vi "AlmostEqual.vi"(0 "VI Reference In":refnum<vi>, 1 "Test Label":string, 2 "delimiter (>>)":string=">>", 3 "Assert Only? (F)":bool, 5 "Control Path":string, 7 "Control Value":ext, 9 "Tolerance":ext=0.00000100000000000000000004, 11 "Error In":errorcluster, 12 "Assert Interval(10 ms)":u32=10, 13 "Timeout(5 sec)":dbl=5.0, 14 "Use Percentage of X (F)":bool) -> (4 "VI Reference Out":refnum<vi>, 6 "Asserted Value":ext, 15 "Error Out":errorcluster)   [LabVIEW 2016, in "Drona.lvlib" / "AssertControlValue.lvlib"]
doc: "Asserts if the numeric values of controls are almost equal.\n\nThe input control name is given as a string , incase of path, use delimiters inbetween the path.\nThis VI gets the value of the control, untill the value is almost equal to the input value."
uses:
  AssertControlValue.lvlib
  Get/GetControlRef/GetControlRefByPath.vi
  <vilib>/addons/_JKI Toolkits/Caraya/classes/Assert/Assert Almost Equal_Float.vi
  <vilib>/addons/_JKI Toolkits/Caraya/classes/Assert/Assert Equal Value_Variant.vi
  <vilib>/addons/_JKI Toolkits/Caraya/classes/Assert/Assert.lvclass
  Get/GetControlRef/GetControlRef.lvlib
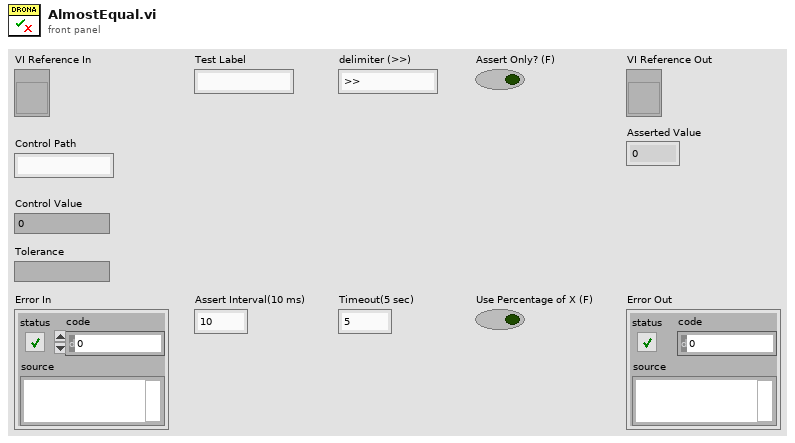
[diagram p1: front panel]
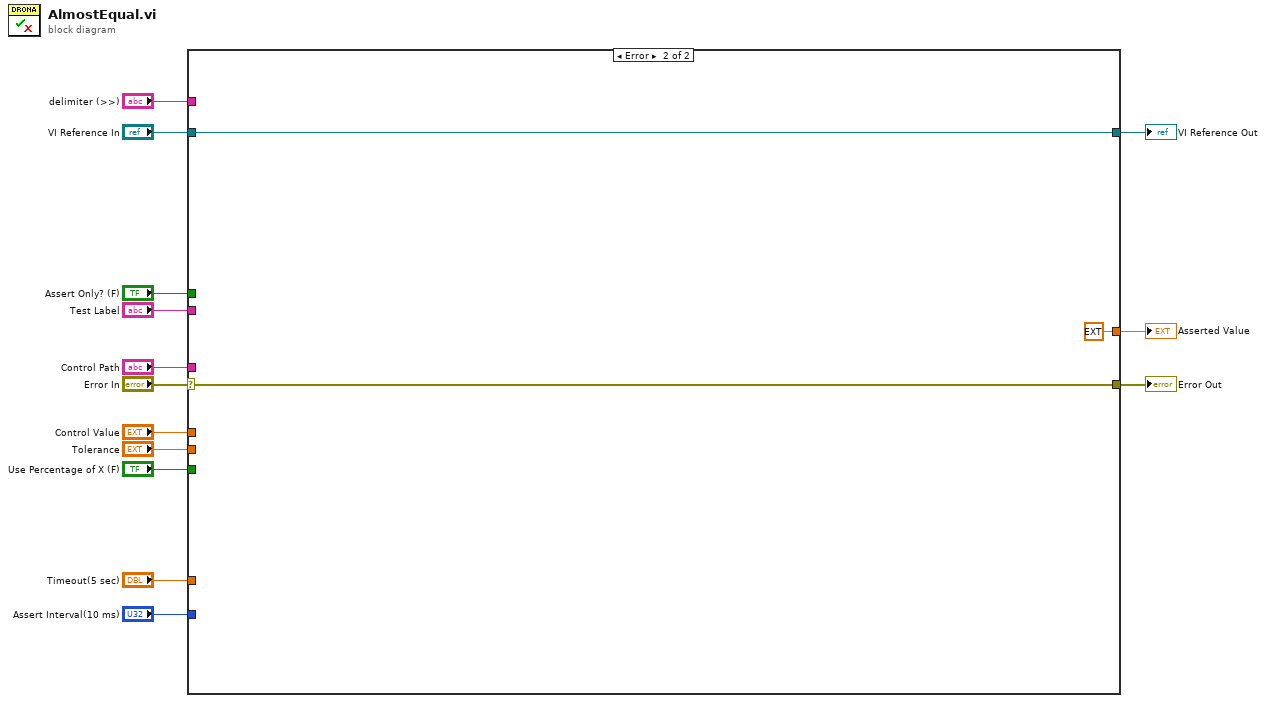
[diagram p0: block diagram]
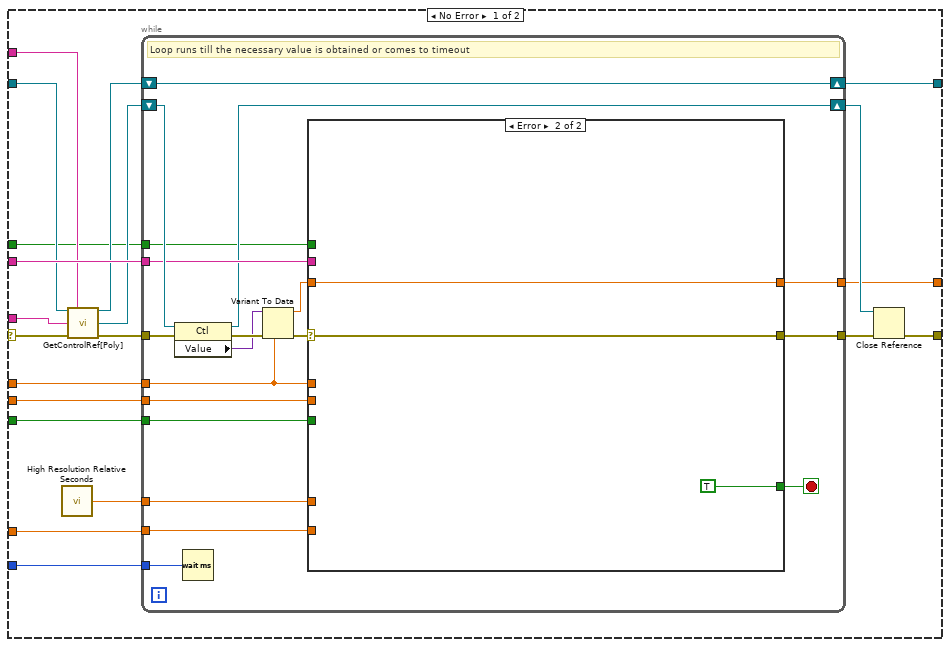
[diagram p2: hidden frame]
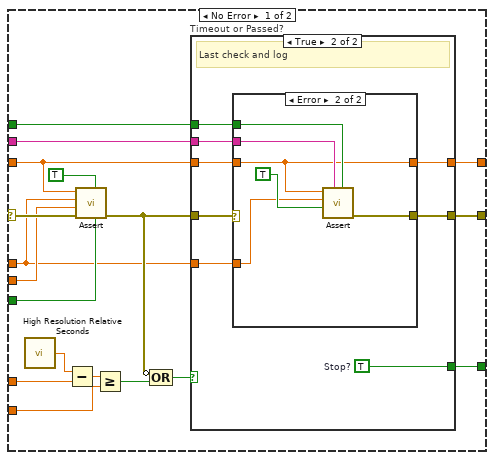
[diagram p3: hidden frame]
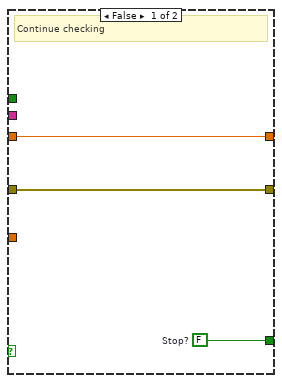
[diagram p4: hidden frame]
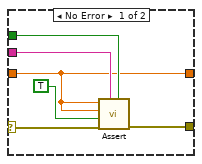
[diagram p5: hidden frame]
diagram:
  n1 = case shown="Error" "Error In" {
    selector: "Error In" -> [w27 w100]
    tunnel: "Timeout(5 sec)" -> [w34 _]
    tunnel: [w33 w99] -> w13
    tunnel: "Control Value" -> [w32 _]
    tunnel: "Tolerance" -> [w31 _]
    tunnel: [w20 w100] -> w10
    tunnel: "Assert Interval(10 ms)" -> [w29 _]
    tunnel: "Test Label" -> [w28 _]
    tunnel: "VI Reference In" -> [w26 w99]
    tunnel: "Control Path" -> [w25 _]
    tunnel: "delimiter (>>)" -> [w18 _]
    tunnel: "Use Percentage of X (F)" -> [w17 _]
    tunnel: "Assert Only? (F)" -> [w16 _]
    tunnel: [w15 ext 0.0 ("Control Value")] -> w1
    frame No Error {
      n2 = call <vilib>:"High Resolution Relative Seconds.vi"() -> ("relative seconds"=w24:dbl)
      n3 = call-poly "GetControlRef[Poly].vi"("VI Reference In"=w26, "delimiter (>>)"=w18, "Control Path"=w25, "error In"=w27) -> ("VI Reference Out"=w22:refnum<vi>, "Ctl Refnum"=w21:refnum<vi>, "error out"=w23:errorcluster)  [unwired: 9 in]
      n4 = while {
        tunnel: w32 -> [w47]
        tunnel: w34 -> [w52]
        tunnel: w24 -> [w53]
        tunnel: w23 -> [w45]
        tunnel: [w50] -> w30
        tunnel: w31 -> [w48]
        tunnel: w29 -> [w36]
        tunnel: w28 -> [w40]
        shift-right: [w43] -> w33
        shift-left: w22 -> [w43]
        shift-right: [w39] -> w19
        shift-left: w21 -> [w44]
        tunnel: w17 -> [w38]
        tunnel: w16 -> [w37]
        tunnel: [w35] -> w15
        stop <- w51 stop-if-true
        # "Loop runs till the necessary value is obtained or comes to timeout"
        n5 = property class="Ctl"(reference=w44, error in=w45) -> (reference out=w39:refnum<vi>, error out=w49:errorcluster, "Value"=w42:variant)
        n6 = Wait (ms)(milliseconds to wait=w36) -> ()  [unwired: 1 out]
        n7 = Variant To Data(error in=w49, type=w47, Variant=w42) -> (data=w46:ext, error out=w41:errorcluster)
        n8 = case shown="Error" w41 {
          selector: w41 -> [w67 w97]
          tunnel: w53 -> [w71 _]
          tunnel: w52 -> [w68 _]
          tunnel: [w61 TRUE] -> w51
          tunnel: [w62 w97] -> w50
          tunnel: w48 -> [w66 _]
          tunnel: w47 -> [w55 _]
          tunnel: w46 -> [w63 w95]
          tunnel: w40 -> [w65 _]
          tunnel: w38 -> [w60 _]
          tunnel: w37 -> [w56 _]
          tunnel: [w54 w95] -> w35
          frame No Error {
            n9 = call <vilib>:"High Resolution Relative Seconds.vi"() -> ("relative seconds"=w70:dbl)
            n10 = Subtract(x=w70, y=w71) -> (x-y=w69:dbl)
            n11 = call-poly <vilib>:"Assert.vi"("Use Percentage of X (F)"=w60, "Assert Only? (F)"=TRUE, "error in (no error)"=w67, "Tolerance"=w66, "Y"=w55, "X"=w63) -> ("error out"=w59:errorcluster)  [unwired: 4 in, 1 out]
            n12 = Greater Or Equal?(x=w69, y=w68) -> (x >= y?=w58:bool)
            n13 = Compound Arithmetic op=OR(invert w59, w58) -> (w57:bool)
            n14 = case "Timeout or Passed?" shown="True" w57 {
              tunnel: w59 -> [w74 w78]
              tunnel: w63 -> [w72 w81]
              tunnel: w65 -> [_ w82]
              tunnel: [w74 w77] -> w62
              tunnel: [w73 w80] -> w61
              tunnel: w56 -> [_ w79]
              tunnel: w55 -> [_ w76]
              tunnel: [w72 w75] -> w54
              frame False {
                w73 = FALSE  # Stop?
                # "Continue checking"
              }
              frame True {
                w80 = TRUE  # Stop?
                # "Last check and log"
                n15 = case shown="Error" w78 {
                  selector: w78 -> [w85 _]
                  tunnel: w82 -> [w88 w94]
                  tunnel: w81 -> [w83 w89]
                  tunnel: w79 -> [w87 w93]
                  tunnel: [w84 w92] -> w77
                  tunnel: w76 -> [_ w90]
                  tunnel: [w83 w89] -> w75
                  frame No Error {
                    n16 = call-poly <vilib>:"Assert.vi"("Assert Only? (F)"=w87, "Label"=w88, "error in (no error)"=w85, "Register with caller test (F)"=TRUE, "Y"=w83, "X"=w83) -> ("error out"=w84:errorcluster)  [unwired: 4 in, 1 out]
                  }
                  frame Error {
                    n17 = call-poly <vilib>:"Assert.vi"("Assert Only? (F)"=w93, "Label"=w94, "Register with caller test (F)"=TRUE, "Y"=w90, "X"=w89) -> ("error out"=w92:errorcluster)  [unwired: 5 in, 1 out]
                  }
                }
              }
            }
          }
          frame Error {
          }
        }
      }
      n18 = Close Reference(reference=w19, error in (no error)=w30) -> (error out=w20:errorcluster)
    }
    frame Error {
    }
  }
  "Error Out" <- w10
  "VI Reference Out" <- w13
  "Asserted Value" <- w1
